vi "configure.vi"(8 "error in (no error)":errorcluster, 11 "DL090216Display in":refnum<class "DisplayDL090216.lvclass">) -> (0 "error out":errorcluster, 3 "DL090216Display out":refnum<class "DisplayDL090216.lvclass">)   [LabVIEW 2010, in "DisplayDL090216.lvclass"]
uses:
  DisplayDL090216.lvclass
  common/clusters/plugin_specification.ctl
  <vilib>/Utility/miscctls.llb/LVPointTypeDef.ctl
  DisplayDL090216.lvclass/DisplayDL090216.ctl
  ImageProcessor/ImageProcessorDL090216RangeOffset/ImageProcessorDL090216RangeOffset/ImageProcessorDL090216RangeOffset.lvclass
  ImageProcessor/GenericImageProcessor/GenericImageProcessor/GenericImageProcessor.lvclass
  common/classes/ErrorController/ErrorController/class_data.vi
  common/classes/GenericComponent/GenericComponent/GenericComponent.lvclass
  common/classes/ErrorController/ErrorController/ErrorController.lvclass
panel:
  out "Configuration":string
  in  "cancel":bool
  in  "save":bool
  in  "Tab Control":T1(tab)
  in  "Number of channels":i32 min=0 max=10
  in  "range/offset processor configuration":string(combo) caption="configuration"
  in  "editImageProcessorListButton":bool
  in  "enable histograms":bool=TRUE
  in  "channel_3_max":dbl=65535.0 caption="to"
  in  "channel_3_min":dbl caption="channel 3"
  in  "channel_2_max":dbl=65535.0 caption="to"
  in  "channel_2_min":dbl caption="channel 2"
  in  "channel_1_max":dbl=65535.0 caption="to"
  in  "channel_1_min":dbl caption="channel 1"
  in  "autoscale histogram":bool=TRUE
  # "Configure DisplayDL090216"
  # "The task of the DisplayDL090216 component is to display images to the user."
  # "Specify how many of the acquired channels will be visible on the display. \n\nImportant: Note that this number can be smaller than the actual number of channels acquired because you might not want to display certain channels (e.g., scanner position feedback channels). By displaying less channels, the computational load is reduced."
  # "Range-and-offset processor"
  # "The range-and-offset processor adjusts range and offset of the images displayed. You have to configure it individually and then select its configuration file name here."
  # "Here, you can specify additional imageProcessors that will further modify the images before display.\n\nImportant: Note that these modifications do not have impact on how images that are stored to disk."
  # "Here, you can specify if the histograms are shown and what the scaling is.\n\nFor high speed imaging, where images are shown at high rates (>15 fps) it might give speed advantages. \n\nManual range can be practical for users who use always the same pixel dwell times"
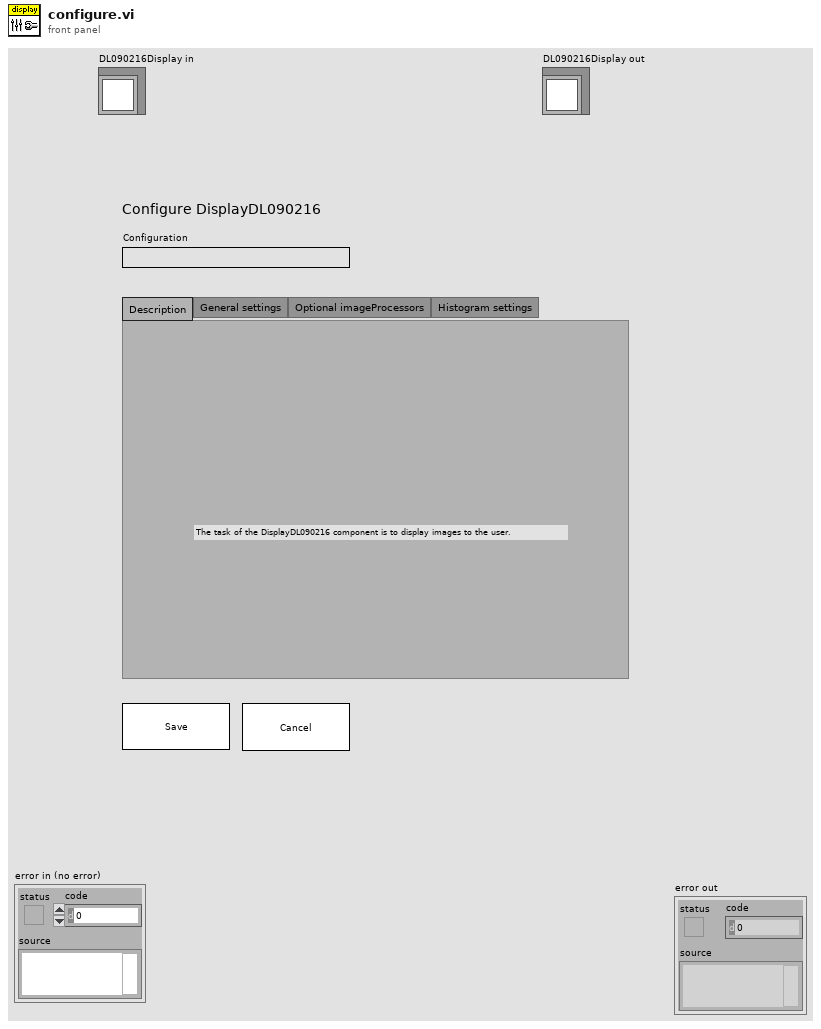
[diagram p1: front panel]
types:
  T1 = enum32{"Description", "General settings", "Optional imageProcessors", "Histogram settings"}
  T2 = typedef "plugin_specification.ctl" = cluster{"class path":string, "configuration":string, "label":string, "settings name":string}
  T3 = typedef "LVPointTypeDef.ctl" = cluster{"Horizontal":i16, "Vertical":i16}
  T4 = enum8{"Enabled", "Disabled", "Disabled and Grayed Out"}
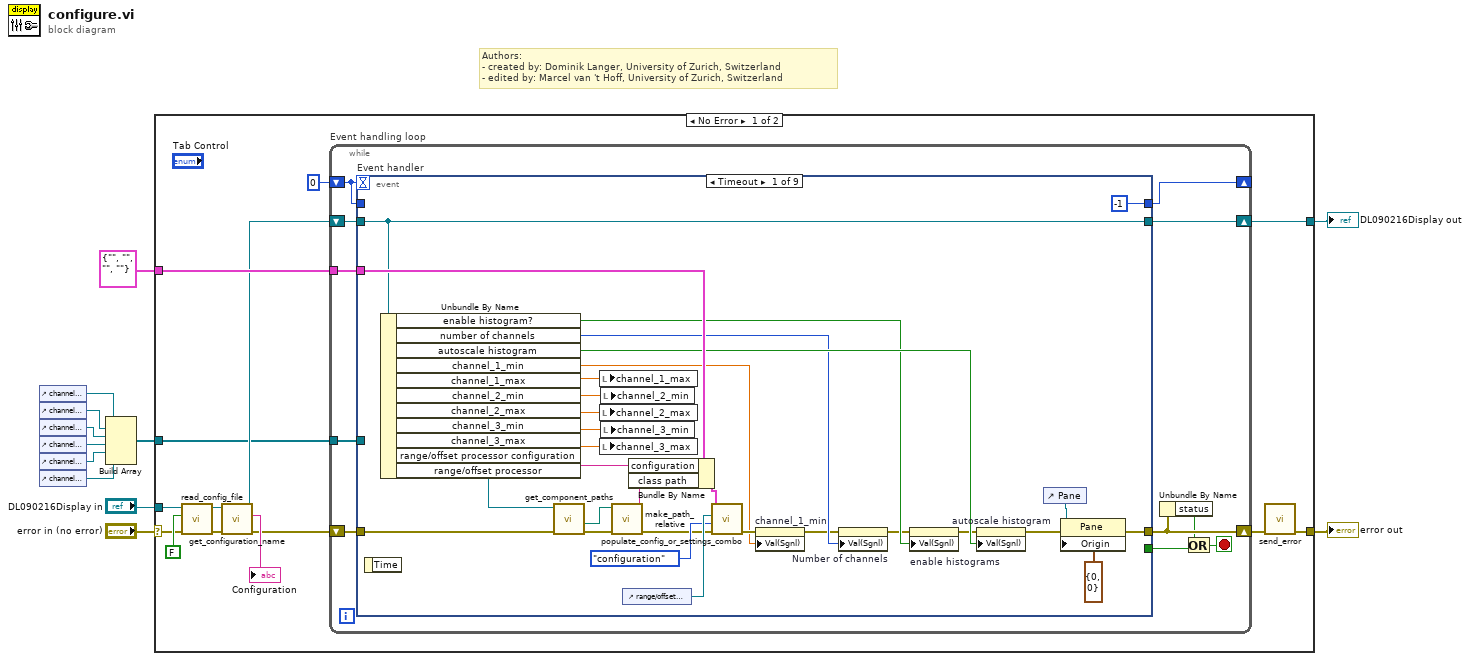
[diagram p0: block diagram]
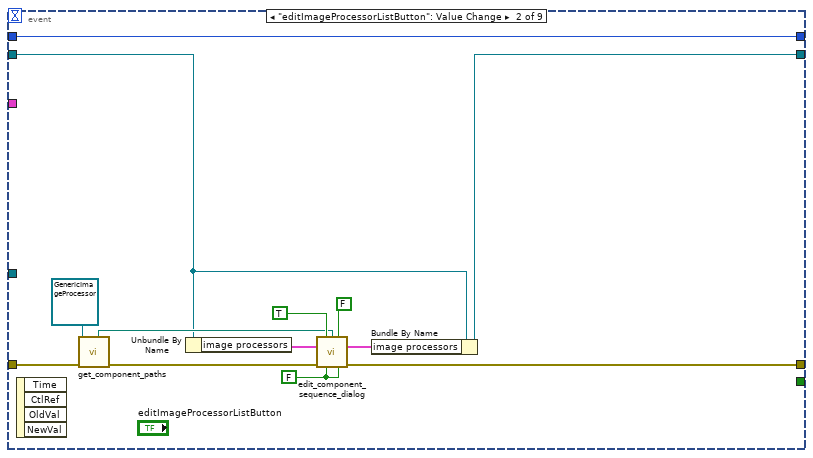
[diagram p2: hidden frame]
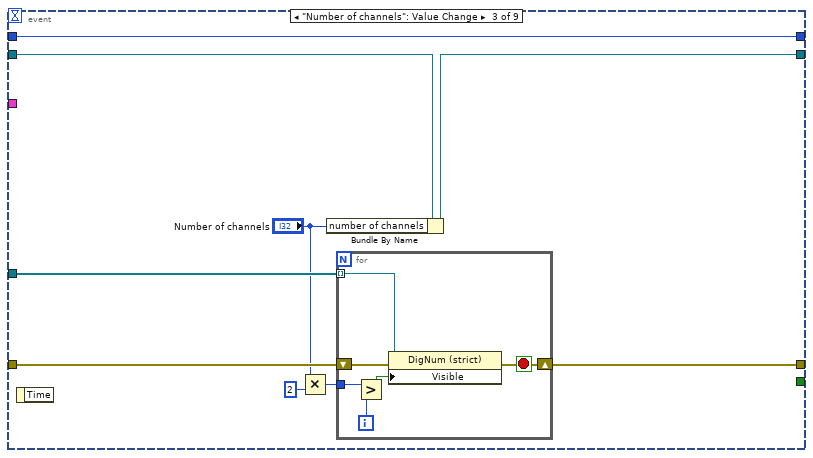
[diagram p3: hidden frame]
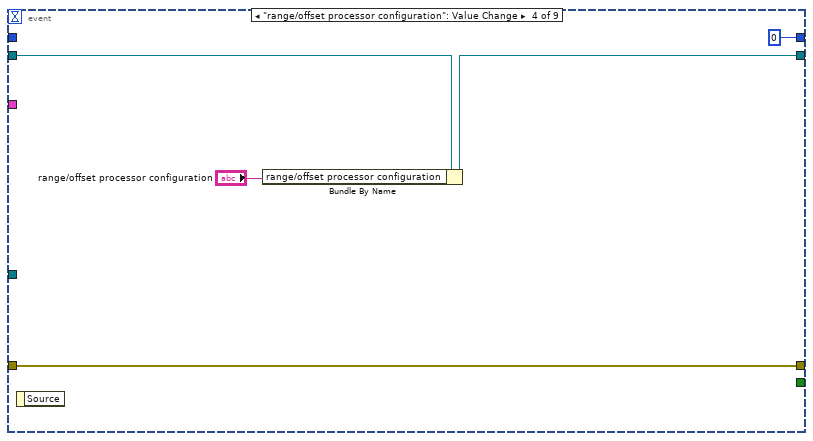
[diagram p4: hidden frame]
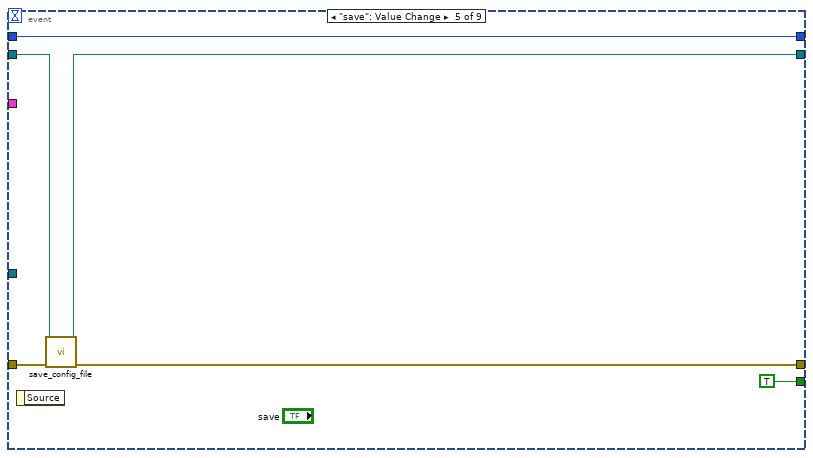
[diagram p5: hidden frame]
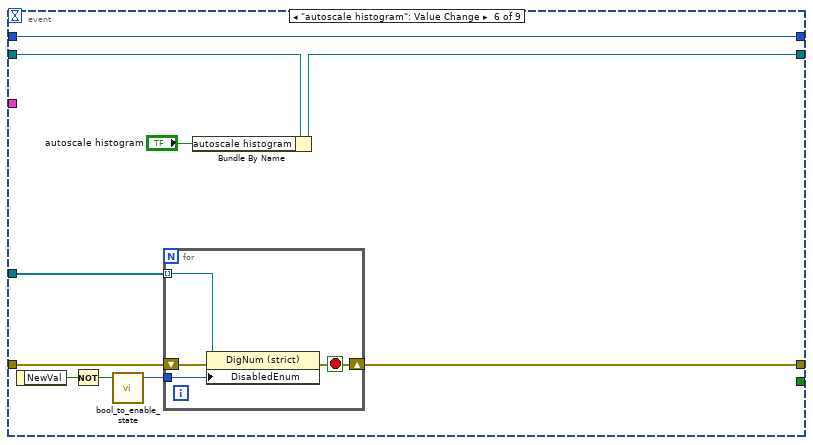
[diagram p6: hidden frame]
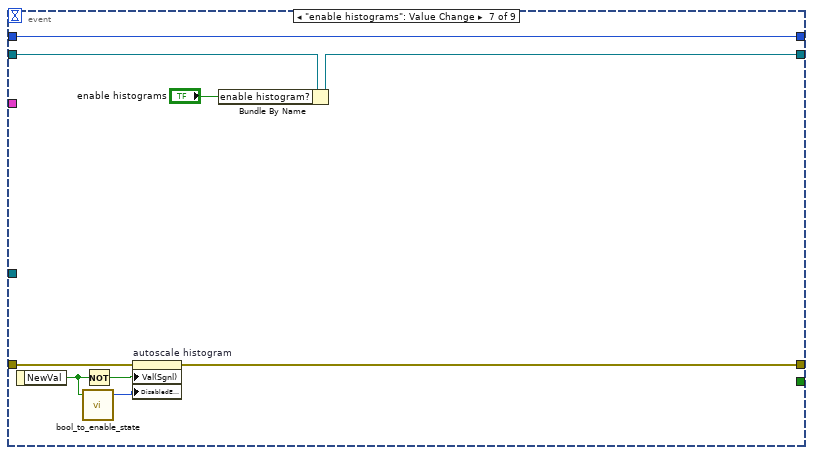
[diagram p7: hidden frame]
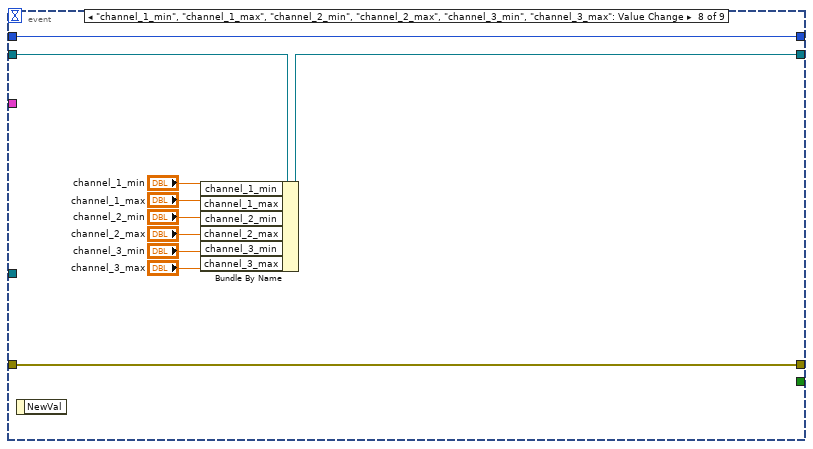
[diagram p8: hidden frame]
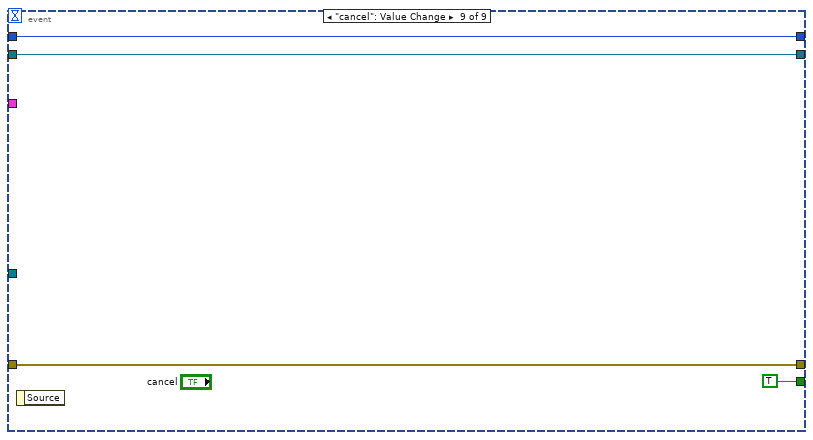
[diagram p9: hidden frame]
diagram:
  # "Authors: \n- created by: Dominik Langer, University of Zurich, Switzerland\n- edited by: Marcel van 't Hoff, University of Zurich, Switzerland"
  n1 = control-ref of="channel_1_min"() -> (w7:refnum<vi>)
  n2 = control-ref of="channel_1_max"() -> (w6:refnum<vi>)
  n3 = control-ref of="channel_2_min"() -> (w5:refnum<vi>)
  n4 = control-ref of="channel_2_max"() -> (w4:refnum<vi>)
  n5 = control-ref of="channel_3_min"() -> (w3:refnum<vi>)
  n6 = control-ref of="channel_3_max"() -> (w2:refnum<vi>)
  n7 = Build Array(w7, w6, w5, w4, w3, w2) -> (w1:refnum<vi>[])
  n8 = case shown="No Error" "error in (no error)" {
    selector: "error in (no error)" -> [w24 w145]
    tunnel: [w16 w145] -> w11
    tunnel: [w22 w144] -> w9
    tunnel: "DL090216Display in" -> [w25 w144]
    tunnel: T2 {"class path"="", "configuration"="", "label"="", "settings name"=""} ("configuration data.clock") -> [w21 _]
    tunnel: w1 -> [w14 _]
    frame No Error {
      n9 = call-dynamic "read_config_file.vi"("error in (no error)"=w24, "force load?"=FALSE, "GenericPlugin in"=w25) -> ("error out"=w13:errorcluster, "GenericPlugin out"=w20:refnum<class "DisplayDL090216.lvclass">)  [unwired: 7 out]
      n10 = call "get_configuration_name.vi"("error in (no error)"=w13, "GenericPlugin.lvclass in"=w20) -> ("error out"=w17:errorcluster, "configuration name"=→"Configuration":string, "GenericPlugin.lvclass out"=w19:refnum<class "DisplayDL090216.lvclass">)  [unwired: 7 in]
      n11 = while "Event handling loop" {
        shift-right: [w33] -> _
        shift-left: 0 -> [w37]
        shift-right: [w35] -> w22
        shift-left: w19 -> [w36]
        tunnel: w21 -> [w34]
        tunnel: w14 -> [w28]
        shift-right: [w32] -> w15
        shift-left: w17 -> [w27]
        stop <- w29 stop-if-true
        n12 = event "Event handler" shown="[0] Timeout" {
          selector: _ -> [_ _ _ _ _ _ _ _ _]
          dyn-events: _ -> [_ _ _ _ _ _ _ _ _]
          timeout: w37 -> [_ _ _ _ _ _ _ _ _]
          tunnel: w27 -> [w60 w73 w86 w100 w104 w114 w128 w139 w143]
          tunnel: [w43 w79 w85 w100 w103 w113 w127 w139 w143] -> w32
          tunnel: [-1 w80 w89 0 w106 w116 w129 w138 w142] -> w33
          tunnel: w37 -> [_ w80 w89 _ w106 w116 w129 w138 w142]
          tunnel: w36 -> [w61 w68 w88 w99 w101 w111 w123 w131 w141]
          tunnel: [w61 w76 w87 w98 w102 w110 w122 w130 w141] -> w35
          tunnel: w34 -> [w66 _ _ _ _ _ _ _ _]
          tunnel: [_ _ _ _ TRUE _ _ _ TRUE] -> w31
          tunnel: w28 -> [_ _ w84 _ _ w115 _ _ _]
          event Timeout {
            n13 = event-data() -> ()  [unwired: 2 out]
            n14 = Unbundle By Name(w61) -> ("enable histogram?"=w46:bool, "number of channels"=w47:i32, "autoscale histogram"=w48:bool, "channel_1_min"=w49:dbl, "channel_1_max"=w51:dbl, "channel_2_min"=w52:dbl, "channel_2_max"=w53:dbl, "channel_3_min"=w54:dbl, "channel_3_max"=w55:dbl, "range/offset processor configuration"=w65:string, "range/offset processor"=w59:refnum<class "ImageProcessorDL090216RangeOffset.lvclass">)
            n15 = call-dynamic "get_component_paths.vi"("error in (no error)"=w60, "GenericComponent in"=w59) -> ("error out"=w42:errorcluster, "component class path"=w58:path)  [unwired: 4 in, 4 out]
            n16 = local write "channel_1_max"(w51) -> ()
            n17 = local write "channel_2_max"(w53) -> ()
            n18 = local write "channel_3_max"(w55) -> ()
            n19 = local write "channel_2_min"(w52) -> ()
            n20 = local write "channel_3_min"(w54) -> ()
            n21 = call "make_path_relative.vi"("error in (no error)"=w42, "absolute path"=w58) -> ("error out"=w56:errorcluster, "relative path"=w57:string)  [unwired: 8 in]
            n22 = control-ref of="range/offset processor configuration"() -> (w64:refnum<vi>)
            n23 = Bundle By Name(cluster=w66, "configuration"=w65, "class path"=w57) -> (w63:T2)
            n24 = call "populate_config_or_settings_combo.vi"("error in (no error)"=w56, "type"=enum16{"configuration", "settings"}."configuration", "combo-box reference"=w64, "plug-in specification"=w63) -> ("error out"=w50:errorcluster)  [unwired: 7 in]
            n25 = property on="channel_1_min" class="DigNum (strict)"(error in=w50, "Val(Sgnl)"=w49) -> (error out=w41:errorcluster)  [unwired: 1 in, 1 out]
            n26 = property on="Number of channels" class="DigNum (strict)"(error in=w41, "Val(Sgnl)"=w47) -> (error out=w40:errorcluster)  [unwired: 1 in, 1 out]
            n27 = property on="enable histograms" class="Bool (strict)"(error in=w40, "Val(Sgnl)"=w46) -> (error out=w39:errorcluster)  [unwired: 1 in, 1 out]
            n28 = property on="autoscale histogram" class="Bool (strict)"(error in=w39, "Val(Sgnl)"=w48) -> (error out=w38:errorcluster)  [unwired: 1 in, 1 out]
            n29 = control-ref of="Pane"() -> (w45:refnum<vi>)
            n30 = property class="Pane"(reference=w45, error in=w38, "Origin"=T3 {"Horizontal"=0, "Vertical"=0}) -> (error out=w43:errorcluster)  [unwired: 1 out]
          }
          event "editImageProcessorListButton": Value Change {
            w75 = FALSE ("choose default?")
            n31 = event-data() -> ()  [unwired: 5 out]
            n32 = call-dynamic "get_component_paths.vi"("error in (no error)"=w73, "GenericComponent in"=refnum<class "GenericImageProcessor.lvclass"> refnum ("GenericImageProcessor.lvclass")) -> ("error out"=w72:errorcluster, "component type directory"=w69:path)  [unwired: 4 in, 4 out]
            n33 = Unbundle By Name(w68) -> ("image processors"=w78:T2[])
            n34 = call "edit_component_sequence_dialog.vi"("show configuration?"=TRUE, "default folder path"=w69, "show label?"=FALSE, "component specification list in"=w78, "error in (no error)"=w72, "choose default?"=w75, "show settings?"=w75) -> ("component specification list out"=w77:T2[], "error out"=w79:errorcluster)  [unwired: 6 in, 1 out]
            n35 = Bundle By Name(cluster=w68, "image processors"=w77) -> (w76:refnum<class "DisplayDL090216.lvclass">)
          }
          event "Number of channels": Value Change {
            n36 = event-data() -> ()  [unwired: 2 out]
            n37 = Multiply(x="Number of channels", y=2) -> (x*y=w81:i32)
            n38 = Bundle By Name(cluster=w88, "number of channels"="Number of channels") -> (w87:refnum<class "DisplayDL090216.lvclass">)
            n39 = for {
              tunnel: w84 -> [w95] mode=indexing
              shift-right: [w93] -> w85
              shift-left: w86 -> [w94]
              tunnel: w81 -> [w92]
              i -> [w91]
              stop <- w93 stop-if-true
              n40 = Greater?(x=w92, y=w91) -> (0:w90:bool)
              n41 = property class="DigNum (strict)"(reference=w95, error in=w94, "Visible"=w90) -> (error out=w93:errorcluster)  [unwired: 1 out]
            }
          }
          event "range/offset processor configuration": Value Change {
            n42 = event-data() -> ()  [unwired: 2 out]
            n43 = Bundle By Name(cluster=w99, "range/offset processor configuration"="range/offset processor configuration") -> (w98:refnum<class "DisplayDL090216.lvclass">)
          }
          event "save": Value Change {
            n44 = event-data() -> ()  [unwired: 2 out]
            n45 = call-dynamic "save_config_file.vi"("error in (no error)"=w104, "GenericPlugin in"=w101) -> ("error out"=w103:errorcluster, "GenericPlugin out"=w102:refnum<class "DisplayDL090216.lvclass">)  [unwired: 2 in, 6 out]
          }
          event "autoscale histogram": Value Change {
            n46 = event-data() -> ("NewVal"=w109:bool)  [unwired: 1 out]
            n47 = Not(x=w109) -> (.not. x?=w108:bool)
            n48 = call "bool_to_enable_state.vi"("boolean in"=w108) -> ("enabled status out"=w107:T4)  [unwired: 4 in]
            n49 = for {
              tunnel: w115 -> [w120] mode=indexing
              tunnel: w107 -> [w118]
              shift-right: [w117] -> w113
              shift-left: w114 -> [w119]
              stop <- w117 stop-if-true
              n50 = property class="DigNum (strict)"(reference=w120, error in=w119, "DisabledEnum"=w118) -> (error out=w117:errorcluster)  [unwired: 1 out]
            }
            n51 = Bundle By Name(cluster=w111, "autoscale histogram"="autoscale histogram") -> (w110:refnum<class "DisplayDL090216.lvclass">)
          }
          event "enable histograms": Value Change {
            n52 = event-data() -> ("NewVal"=w125:bool)  [unwired: 1 out]
            n53 = call "bool_to_enable_state.vi"("boolean in"=w125) -> ("enabled status out"=w124:T4)  [unwired: 4 in]
            n54 = Not(x=w125) -> (.not. x?=w126:bool)
            n55 = property on="autoscale histogram" class="Bool (strict)"(error in=w128, "Val(Sgnl)"=w126, "DisabledEnum"=w124) -> (error out=w127:errorcluster)  [unwired: 1 in, 1 out]
            n56 = Bundle By Name(cluster=w123, "enable histogram?"="enable histograms") -> (w122:refnum<class "DisplayDL090216.lvclass">)
          }
          event "channel_1_min", "channel_1_max", "channel_2_min", "channel_2_max", "channel_3_min", "channel_3_max": Value Change {
            n57 = event-data() -> ()  [unwired: 2 out]
            n58 = Bundle By Name(cluster=w131, "channel_1_min"="channel_1_min", "channel_1_max"="channel_1_max", "channel_2_min"="channel_2_min", "channel_2_max"="channel_2_max", "channel_3_min"="channel_3_min", "channel_3_max"="channel_3_max") -> (w130:refnum<class "DisplayDL090216.lvclass">)
          }
          event "cancel": Value Change {
            n59 = event-data() -> ()  [unwired: 2 out]
          }
        }
        n60 = Unbundle By Name(w32) -> ("status"=w30:bool)
        n61 = Or(x=w30, y=w31) -> (x .or. y?=w29:bool)
      }
      n62 = call "send_error.vi"("error in (no error)"=w15) -> ("error out"=w16:errorcluster)  [unwired: 10 in]
    }
    frame Error {
    }
  }
  "error out" <- w11
  "DL090216Display out" <- w9
